vi "Refresh Skipfire Listbox.vi"(7 "ChannelNames":string[](array[string]), 8 "IRQ Settings Array":T1[](array[typedef]), 11 "IRQ Listbox Refnum":refnum<vi>) -> ()   [LabVIEW 2016]
uses:
  <vilib>/Powertrain Controls/Device Drivers/DCM/Skip Fire/RT/Skip Fire Setup.ctl
  <vilib>/Powertrain Controls/Device Drivers/DCM/Skip Fire/RT/DCM - RT - Skip Fire.lvlib
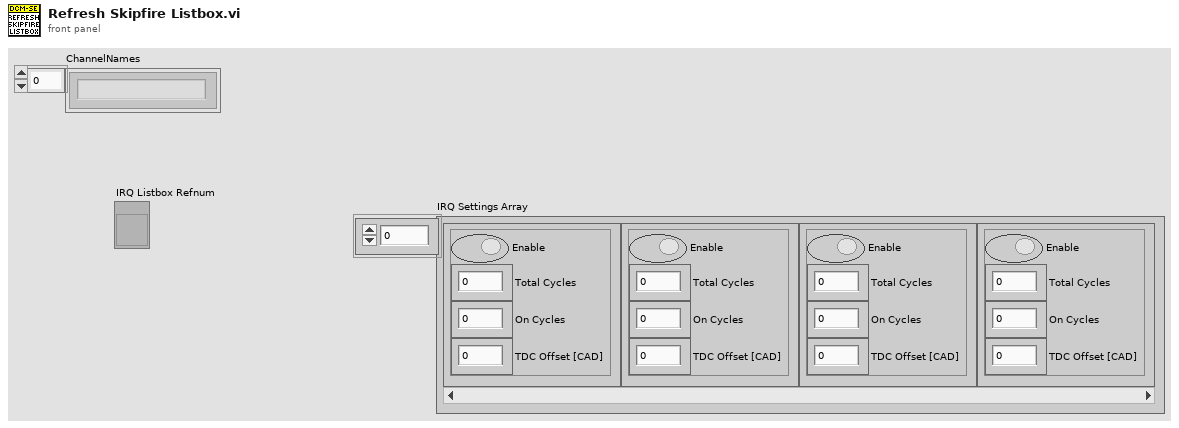
[diagram p1: front panel]
types:
  T1 = typedef "DCM - RT - Skip Fire.lvlib/Skip Fire Setup.ctl" = cluster{"Enable":bool, "Total Cycles":u8, "On Cycles":u8, "TDC Offset [CAD]":sgl}
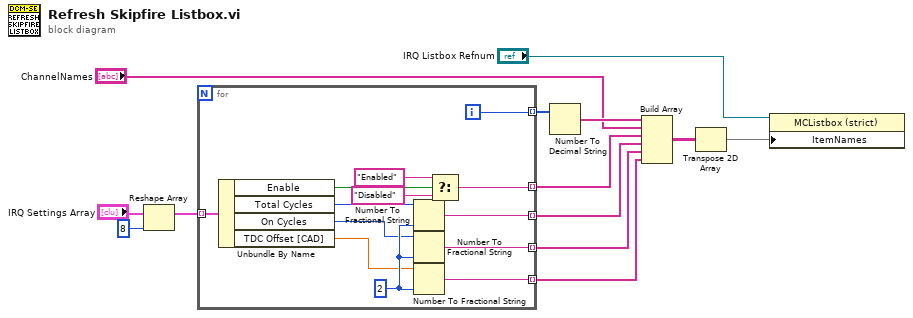
[diagram p0: block diagram]
diagram:
  n1 = Reshape Array("IRQ Settings Array", 8) -> (w11:T1[])
  n2 = for {
    tunnel: w11 -> [w26] mode=indexing
    tunnel: [w14] -> w9 mode=indexing
    tunnel: [w22] -> w5 mode=indexing
    tunnel: [w20] -> w4 mode=indexing
    tunnel: [w16] -> w3 mode=indexing
    tunnel: [w15] -> w2 mode=indexing
    i -> [w14]
    w19 = i16 2 ("precision (6)")
    n3 = Unbundle By Name(w26) -> ("Enable"=w25:bool, "Total Cycles"=w21:u8, "On Cycles"=w18:u8, "TDC Offset [CAD]"=w17:sgl)
    n4 = Number To Fractional String(number=w21, precision (6)=w19) -> (F-format string=w20:string)  [unwired: 2 in]
    n5 = Number To Fractional String(number=w18, precision (6)=w19) -> (F-format string=w16:string)  [unwired: 2 in]
    n6 = Number To Fractional String(number=w17, precision (6)=w19) -> (F-format string=w15:string)  [unwired: 2 in]
    n7 = Select(t="Enabled", s=w25, f="Disabled") -> (s? t:f=w22:string)
  }
  n8 = Number To Decimal String(number=w9) -> (decimal integer string=w10:string[])  [unwired: 1 in]
  n9 = Build Array(w10, "ChannelNames", w5, w4, w3, w2) -> (w13:string[][])
  n10 = Transpose 2D Array(2D array=w13) -> (transposed array=w8:string[][])
  n11 = property on="Property Node" class="MCListbox (strict)"(reference="IRQ Listbox Refnum", "ItemNames"=w8) -> ()  [unwired: 1 in, 2 out]
